vi "UPRESULT.vi"(0 "DEVICE_ID":string, 5 "USER_ID":string, 7 "CODE_ID":string, 9 "RESULT_VALUE":string, 11 "错误输入":errorcluster) -> (15 "error out":errorcluster)   [LabVIEW 2020]
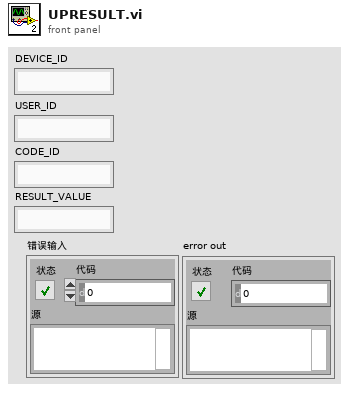
[diagram p1: front panel]
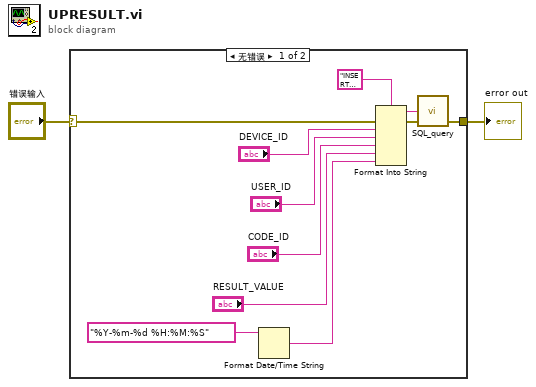
[diagram p0: block diagram]
diagram:
  n1 = case shown="无错误" "错误输入" {
    selector: "错误输入" -> [w3 w14]
    tunnel: [w4 w14] -> w1
    frame No Error {
      n2 = Format Date/Time String(time format string (%c)="%Y-%m-%d %H:%M:%S" ("时间格式字符串(%c)")) -> (date/time string=w11:string)  [unwired: 2 in]
      n3 = Format Into String(format string="INSERT INTO [dbo].[Result] ( [DEVICE_ID], [USER_ID], [CODE_ID], [RESULT_VALUE], [RESULT_TIME] ) \nVALUES\n\t( %s, %s, %s, N'%s', '%s' ) ", error in=w3, "DEVICE_ID", "USER_ID", "CODE_ID", "RESULT_VALUE", w11) -> (resulting string=w13:string, error out=w12:errorcluster)  [unwired: 1 in]
      n4 = call "SQL_query.vi"("error in (no error)"=w12, "SQL query"=w13) -> ("error out"=w4:errorcluster)  [unwired: 2 in, 1 out]
    }
    frame Error {
    }
  }
  "error out" <- w1
